vi "UI.Stream.Enable.vi"(8 "error in (no error)":errorcluster, 11 "State Variables in":T1={"UI.Refs"={"Cmd"=refnum, "Success?"=refnum, "VeriStandError"=refnum, "CAN Connected?"=refnum, "DTC"=refnum, "Status"=refnum, "Failure"=refnum, "Override Byte Lengths"=refnum, "Response Required?"=refnum, "Send"=refnum, "Clear"=refnum, "Send Raw"=refnum, "Read DTCs"=refnum, "Raw Cmd"=refnum, "Extension"=refnum, "Mode"=refnum, "Mask"=refnum, "Hex"=refnum, "Raw Resp"=refnum, "Raw Error Byte"=refnum, "Raw VeriStand Error"=refnum, "DTCs"=refnum, "Time Stamp"=refnum, "Device"=refnum, "Pause"=refnum, "Table Control"=refnum, "Sort By ID"=refnum, "Streaming Connected"=refnum, "Enable Stream"=refnum, "CAN State"=refnum, "Direction Filter"=refnum, "Type Filter"=refnum, "Clear History"=refnum, "Filter IDs"=refnum, "Filter Location"=refnum, "Reset Filter"=refnum, "Log"=refnum}, "Data.PreviousValues"=[], "Data.Read"=[], "CachedData.UserEvent"=refnum, "CachedData"={"CD Path"="", "CD IP"=""}, "Addon.Connected?"=FALSE, "NIVS.SysDef"=path "", "NIVS.SysDefRoot"=refnum, "NIVS.Workspace"=refnum, "NIVS.UserEventRefs"={"Event Registration Refnum"=refnum, "SystemChangeEventRef"=refnum, "NIVS.Workspace Event"=refnum}, "NIVS.SystemStateRefs"={"CustDatRef"=refnum, "EvtRef"=refnum, "Target State User Event"=refnum}, "NIVS.LaunchRef"=refnum, "Data.PendingChange?"=FALSE, "Command.Channel"="", "Diagnostic Protocol"=enum."GMLAN", "Channels.Found"=FALSE, "Command.Connect"="", "Mode.Tool?"=FALSE, "Stream.Qs"={"Cmd Q"=refnum, "XNET Frames"=refnum}, "Transport Layer"=enum."Diagnostics on IP"}) -> (0 "error out":errorcluster)   [LabVIEW 2025, in "Diagnostics Workspace Shared.lvlib"]
uses:
  Diagnostics Workspace Shared.lvlib
  Types/Workspace.State.ctl
  Types/UI.Refs.ctl
  Addon/Addon Shared/Types/Command.New.ctl
  SubModules/CAN-Streaming-Support/Source/Addon/Addon Shared/Types/Type Filter.ctl
  <vilib>/NI VeriStand/Display Template Support/DisplayTemplateSupport.llb/enum_Display Template Handler Minimal To Workspace.ctl
  Types/Workspace.SavedState.ctl
  NationalInstruments.VeriStand.SystemStorage
  <vilib>/NI VeriStand/Execution/Workspace/WorkspaceAPI.ctl
  NationalInstruments.VeriStand.ClientAPI
  <vilib>/NI VeriStand/Display Template Support/DisplayTemplateSupport.llb/enum_Display Template Handler Minimal To Widget Msg.ctl
  <vilib>/NI VeriStand/Execution/Workspace/SystemStateRegEventRef.ctl
  <vilib>/NI VeriStand/Execution/Workspace/Target State Info.ctl
  <vilib>/NI VeriStand/Execution/Workspace/Target State.ctl
  <vilib>/NI VeriStand/Execution/Workspace/SystemStateEventRef.ctl
  Addon/Addon Shared/Types/Protocol.ctl
  SubModules/CAN-Streaming-Support/Source/UIs/Workspace Shared/Types/Host Stream Queue Refs.ctl
  SubModules/CAN-Streaming-Support/Source/UIs/Workspace Shared/Types/Host Stream Queue Type.ctl
  SubModules/CAN-Streaming-Support/Source/UIs/Workspace Shared/Types/Host Stream Queue Command.ctl
  <vilib>/xnet/xnet.llb/XNET Frame CAN.ctl
  <vilib>/xnet/xnet.llb/XNET Frame Type CAN.ctl
  Addon/Addon Shared/Types/Transport.ctl
  <vilib>/Utility/miscctls.llb/LVRowAndColumnUnsignedTypeDef.ctl
  <vilib>/NI VeriStand/Execution/Workspace/NI_VS Workspace ExecutionAPI.lvlib
  Addon/Addon Shared/Diagnostics Addon Shared.lvlib
  SubModules/CAN-Streaming-Support/Source/UIs/Workspace Shared/CAN Stream Support Workspace Shared.lvlib
  SubModules/CAN-Streaming-Support/Source/Addon/Addon Shared/CAN Stream Support Shared.lvlib
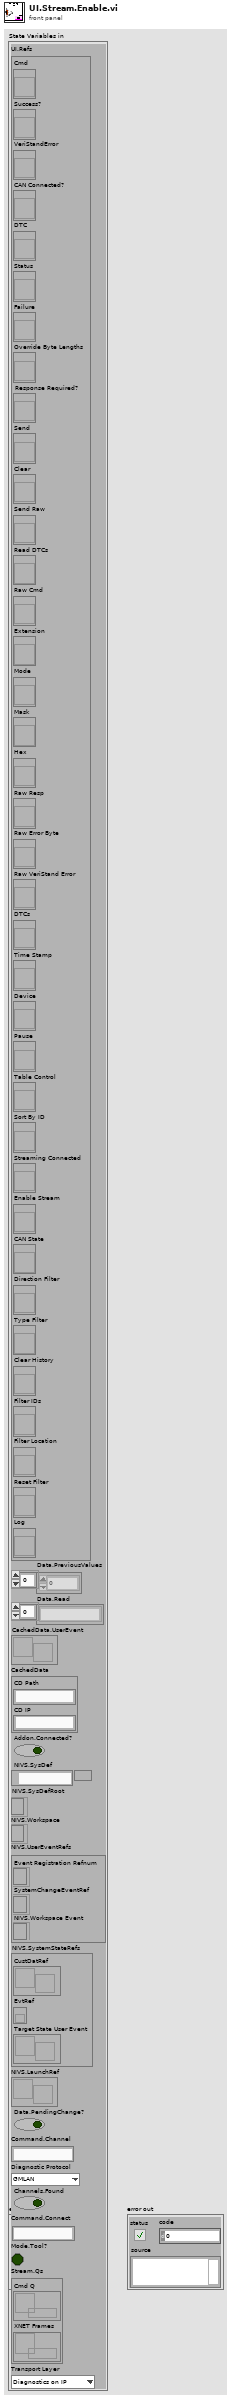
[diagram p1: front panel]
types:
  T1 = typedef "Diagnostics Workspace Shared.lvlib/Workspace.State.ctl" = cluster{"UI.Refs":T2, "Data.PreviousValues":dbl[], "Data.Read":string[], "CachedData.UserEvent":refnum<user-event>, "CachedData":T3, "Addon.Connected?":bool, "NIVS.SysDef":path, "NIVS.SysDefRoot":refnum<k24>, "NIVS.Workspace":T4, "NIVS.UserEventRefs":cluster{"Event Registration Refnum":refnum<event-registration>, "SystemChangeEventRef":T5, "NIVS.Workspace Event":refnum<event-registration>}, "NIVS.SystemStateRefs":T6, "NIVS.LaunchRef":refnum<user-event>, "Data.PendingChange?":bool, "Command.Channel":string, "Diagnostic Protocol":T7, "Channels.Found":bool, "Command.Connect":string, "Mode.Tool?":bool, "Stream.Qs":T8, "Transport Layer":T9}
  T2 = typedef "Diagnostics Workspace Shared.lvlib/UI.Refs.ctl" = cluster{"Cmd":refnum<vi>, "Success?":refnum<vi>, "VeriStandError":refnum<vi>, "CAN Connected?":refnum<vi>, "DTC":refnum<vi>, "Status":refnum<vi>, "Failure":refnum<vi>, "Override Byte Lengths":refnum<vi>, "Response Required?":refnum<vi>, "Send":refnum<vi>, "Clear":refnum<vi>, "Send Raw":refnum<vi>, "Read DTCs":refnum<vi>, "Raw Cmd":refnum<vi>, "Extension":refnum<vi>, "Mode":refnum<vi>, "Mask":refnum<vi>, "Hex":refnum<vi>, "Raw Resp":refnum<vi>, "Raw Error Byte":refnum<vi>, "Raw VeriStand Error":refnum<vi>, "DTCs":refnum<vi>, "Time Stamp":refnum<vi>, "Device":refnum<vi>, "Pause":refnum<vi>, "Table Control":refnum<vi>, "Sort By ID":refnum<vi>, "Streaming Connected":refnum<vi>, "Enable Stream":refnum<vi>, "CAN State":refnum<vi>, "Direction Filter":refnum<vi>, "Type Filter":refnum<vi>, "Clear History":refnum<vi>, "Filter IDs":refnum<vi>, "Filter Location":refnum<vi>, "Reset Filter":refnum<vi>, "Log":refnum<vi>}
  T3 = typedef "Diagnostics Workspace Shared.lvlib/Workspace.SavedState.ctl" = cluster{"CD Path":string, "CD IP":string}
  T4 = typedef "NI_VS Workspace ExecutionAPI.lvlib/WorkspaceAPI.ctl" = refnum<k24>
  T5 = typedef "NI_VS Workspace ExecutionAPI.lvlib/SystemStateRegEventRef.ctl" = refnum<event-registration>
  T6 = typedef "NI_VS Workspace ExecutionAPI.lvlib/SystemStateEventRef.ctl" = cluster{"CustDatRef":refnum<user-event>, "EvtRef":refnum<k27>, "Target State User Event":refnum<user-event>}
  T7 = typedef "Diagnostics Addon Shared.lvlib/Protocol.ctl" = enum16{"GMLAN", "KWP-2000", "UDS", "User-Defined"}
  T8 = typedef "CAN Stream Support Workspace Shared.lvlib/Host Stream Queue Refs.ctl" = cluster{"Cmd Q":refnum<queue>, "XNET Frames":refnum<queue>}
  T9 = typedef "Diagnostics Addon Shared.lvlib/Transport.ctl" = enum16{"ISO TP - Normal Mode", "ISO TP - Mixed Mode", "VW TP 2.0", "Diagnostics on IP", "ISO TP LIN"}
  T10 = enum8{"Enabled", "Disabled", "Disabled and Grayed Out"}
  T11 = typedef "LVRowAndColumnUnsignedTypeDef.ctl" = cluster{"Row":u32, "Column":u32}
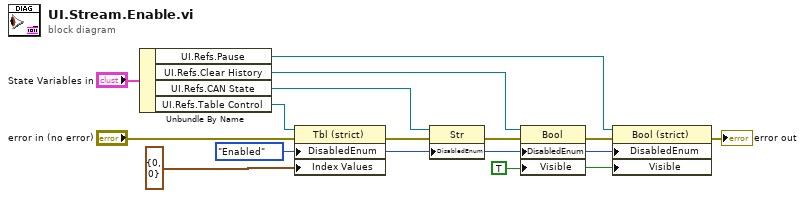
[diagram p0: block diagram]
diagram:
  w1 = TRUE ("Visible")
  w2 = T10."Enabled" ("Disabled")
  n1 = Unbundle By Name("State Variables in") -> ("UI.Refs.Pause"=w3:refnum<vi>, "UI.Refs.Clear History"=w6:refnum<vi>, "UI.Refs.CAN State"=w10:refnum<vi>, "UI.Refs.Table Control"=w13:refnum<vi>)
  n2 = property class="Tbl (strict)"(reference=w13, error in="error in (no error)", "DisabledEnum"=w2, "Index Values"=T11 {"Row"=0, "Column"=0}) -> (error out=w9:errorcluster)  [unwired: 1 out]
  n3 = property class="Str"(reference=w10, error in=w9, "DisabledEnum"=w2) -> (error out=w7:errorcluster)  [unwired: 1 out]
  n4 = property class="Bool"(reference=w6, error in=w7, "DisabledEnum"=w2, "Visible"=w1) -> (error out=w5:errorcluster)  [unwired: 1 out]
  n5 = property class="Bool (strict)"(reference=w3, error in=w5, "DisabledEnum"=w2, "Visible"=w1) -> (error out=→"error out":errorcluster)  [unwired: 1 out]
